vi "AuMT8852B Boot Status Query.vi"(8 "error in (no error)":errorcluster, 11 "VISA session":refnum<visa-resource-name>) -> (0 "error out":errorcluster, 2 "error code":i32, 3 "VISA session out":refnum<visa-resource-name>, 4 "Result":enum16{"Failed", "Passed", "Running"}(ring)=enum."Passed")   [LabVIEW 2017]
doc: "Anritsu MT8852B Bluetooth Tester\n\nReturns the result of the instrument's power-on self-test.\n\nOUTPUTS\nResult - whether the test failed, is still running, or passed."
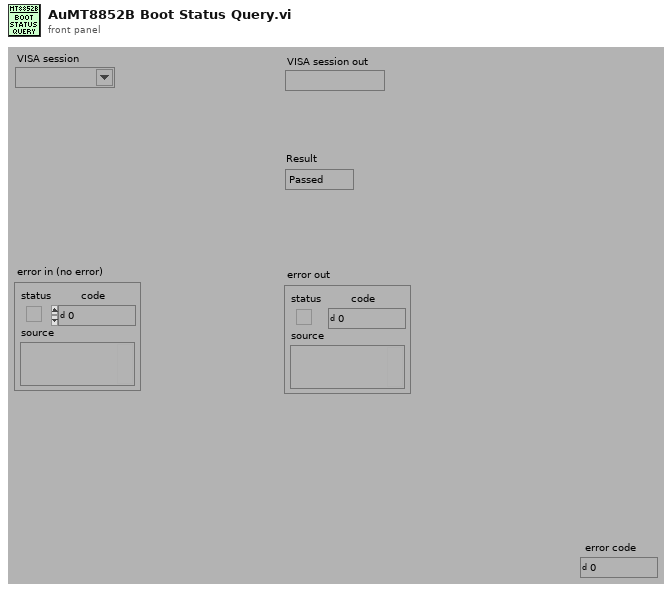
[diagram p1: front panel]
types:
  T1 = enum16{"Simulate", "Range check", "Cache", "Query instrument status"}
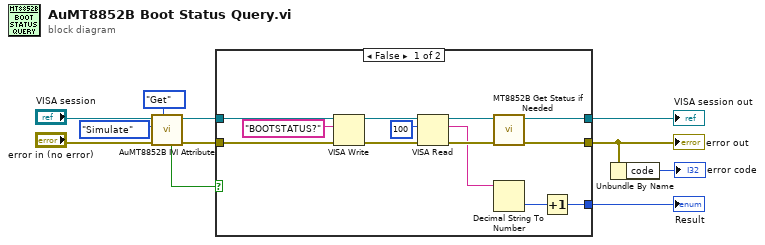
[diagram p0: block diagram]
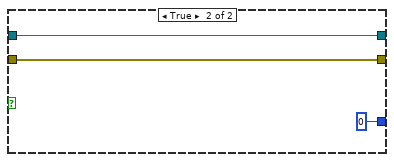
[diagram p2: hidden frame]
diagram:
  n1 = call <instrlib>:"AuMT8852B IVI Attribute.vi"("Set/Get (Set)"=enum16{"Set", "Get"}."Get", "error in (no error)"="error in (no error)", "Flag (Simulate)"=T1."Simulate", "VISA session"="VISA session") -> ("error out"=w7:errorcluster, "VISA session out"=w8:refnum<visa-resource-name>, "Value out"=w3:bool)  [unwired: 5 in]
  n2 = case shown="False" w3 {
    tunnel: [w20 w26] -> w1
    tunnel: [w21 w27] -> w9
    tunnel: w8 -> [w24 w27]
    tunnel: w7 -> [w23 w26]
    tunnel: [w13 0] -> w6
    frame False {
      n3 = VISA Write(VISA resource name=w24, write buffer="BOOTSTATUS?" ("write buffer (\"\")"), error in (no error)=w23) -> (VISA resource name out=w19:refnum<visa-resource-name>, error out=w16:errorcluster)  [unwired: 1 out]
      n4 = VISA Read(VISA resource name=w19, byte count=u32 100 ("byte count (0)"), error in (no error)=w16) -> (VISA resource name out=w15:refnum<visa-resource-name>, read buffer=w12:string, error out=w14:errorcluster)  [unwired: 1 out]
      n5 = call <instrlib>:"MT8852B Get Status if Needed.vi"("error in (no error)"=w14, "VISA session"=w15) -> ("error out"=w20:errorcluster, "VISA session out"=w21:refnum<visa-resource-name>)  [unwired: 8 in]
      n6 = Decimal String To Number(string=w12) -> (number=w22:i32)  [unwired: 2 in, 1 out]
      n7 = Increment(x=w22) -> (x+1=w13:i32)
    }
    frame True {
    }
  }
  "error out" <- w1
  "VISA session out" <- w9
  "Result" <- w6
  n8 = Unbundle By Name(w1) -> ("code"=→"error code":i32)
